vi "ControlRefnumStore__slk_refnum.vi"(6 "cmd (Get)":enum16{"Set", "Get"}(ring)=enum."Get", 8 "error in (no error)":errorcluster, 11 "vi refnum in (use current vi if non-wired)":refnum<vi>) -> (0 "error out":errorcluster, 3 "control refnum array out":refnum<vi>[](array[refnum]))   [LabVIEW 2020, in "REFNUM.lvlib"]
doc: "<b>Refnum Functions:</b>\nReset - Initializes all controls' refnum from current VI to GL.\nGet - Gets all controls's refnum from GL."
uses:
  Library/Refnum.lvlib
panel:
  # "ControlRefnumStore__slk_refnum.vi\n\nNOTICE -- YOU MUST LEAVE THIS NOTICE IN PLACE.\n\nCopyright (c) 2008 Shawn Liu <shawn.liu.cn@gmail.com>\n\nAll rights reserved."
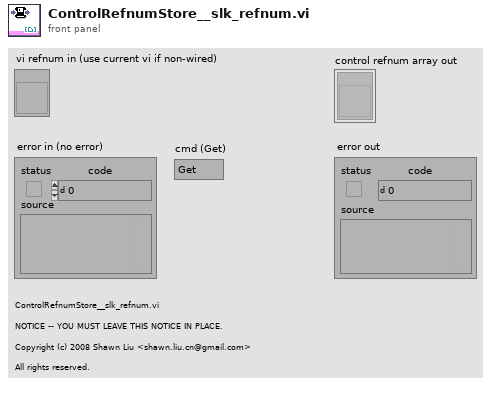
[diagram p1: front panel]
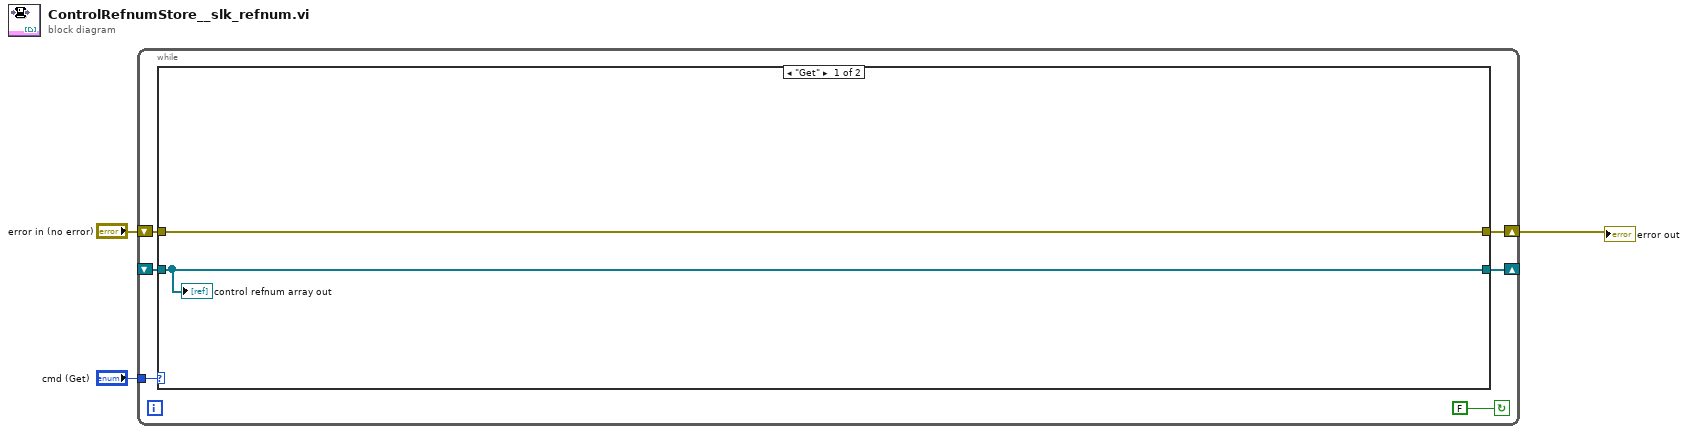
[diagram p0: block diagram]
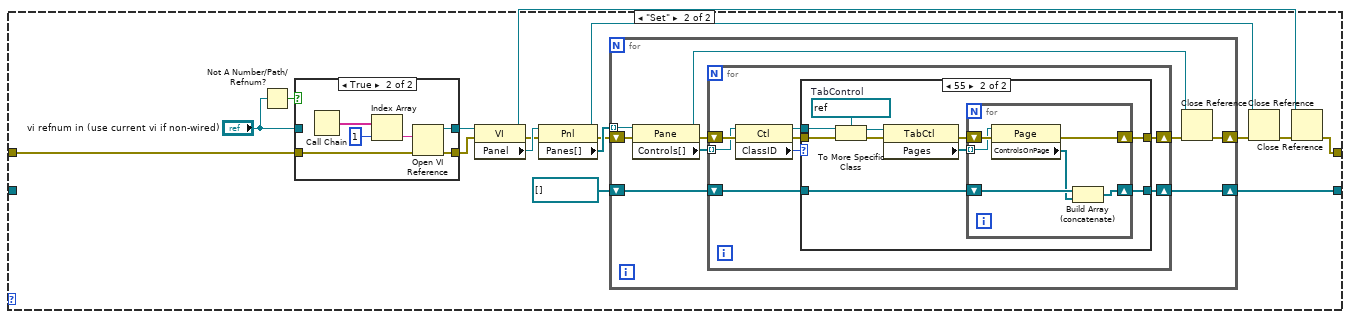
[diagram p2: hidden frame]
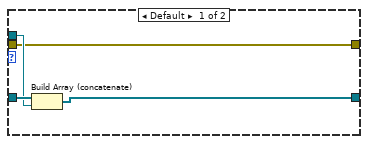
[diagram p4: hidden frame]
diagram:
  n1 = while {
    tunnel: "cmd (Get)" -> [w9]
    shift-right: [w8] -> _
    shift-left: _ -> [w7]
    shift-right: [w5] -> w1
    shift-left: "error in (no error)" -> [w6]
    stop <- FALSE continue-if-true
    n2 = case shown="\"Get\"" w9 {
      tunnel: [w11 w25] -> w8
      tunnel: w7 -> [w11 _]
      tunnel: w6 -> [w10 w21]
      tunnel: [w10 w24] -> w5
      frame "Get" {
        "control refnum array out" <- w11
      }
      frame "Set" {
        n3 = Not A Number/Path/Refnum?(number/path/refnum="vi refnum in (use current vi if non-wired)") -> (NaN/Path/Refnum?=w23:bool)
        n4 = case shown="True" w23 {
          tunnel: [w29 w32] -> w19
          tunnel: [w28 w31] -> w20
          tunnel: w21 -> [w28 w30]
          tunnel: "vi refnum in (use current vi if non-wired)" -> [w29 _]
          frame False {
          }
          frame True {
            n5 = Call Chain() -> (call chain=w35:string[])
            n6 = Index Array(array=w35, index=1) -> (element=w33:string)
            n7 = Open VI Reference(vi path=w33, error in (no error)=w30) -> (vi reference=w32:refnum<vi>, error out=w31:errorcluster)  [unwired: 4 out]
          }
        }
        n8 = property class="VI"(reference=w19, error in=w20) -> (reference out=w12:refnum<vi>, error out=w17:errorcluster, "Panel"=w18:refnum<vi>)
        n9 = property class="Pnl"(reference=w18, error in=w17) -> (reference out=w13:refnum<vi>, error out=w15:errorcluster, "Panes[]"=w16:refnum<vi>[])
        n10 = for {
          tunnel: w16 -> [w44] mode=indexing
          shift-right: [w37] -> w14
          shift-left: w15 -> [w43]
          shift-right: [w41] -> w25
          shift-left: refnum<vi>[] [] -> [w42]
          n11 = property class="Pane"(reference=w44, error in=w43) -> (reference out=w36:refnum<vi>, error out=w39:errorcluster, "Controls[]"=w40:refnum<vi>[])
          n12 = for {
            shift-right: [w45] -> w41
            shift-left: w42 -> [w47]
            tunnel: w40 -> [w51] mode=indexing
            shift-right: [w46] -> w38
            shift-left: w39 -> [w52]
            n13 = property class="Ctl"(reference=w51, error in=w52) -> (reference out=w49:refnum<vi>, error out=w48:errorcluster, "ClassID"=w50:u32)
            n14 = case shown="55" w50 {
              tunnel: w49 -> [w54 w64]
              tunnel: w48 -> [w53 w66]
              tunnel: w47 -> [w56 w59]
              tunnel: [w53 w58] -> w46
              tunnel: [w55 w57] -> w45
              frame Default {
                n15 = Build Array (concatenate)(w56, w54) -> (w55:refnum<vi>[])
              }
              frame 55 {
                w62 = refnum<vi> refnum  # TabControl
                n16 = To More Specific Class(target class=w62, reference=w64, error in=w66) -> (specific class reference=w63:refnum<vi>, error out=w65:errorcluster)
                n17 = property class="TabCtl"(reference=w63, error in=w65) -> (error out=w60:errorcluster, "Pages"=w61:refnum<vi>[])  [unwired: 1 out]
                n18 = for {
                  tunnel: w61 -> [w71] mode=indexing
                  shift-right: [w68] -> w57
                  shift-left: w59 -> [w70]
                  shift-right: [w67] -> w58
                  shift-left: w60 -> [w72]
                  n19 = property class="Page"(reference=w71, error in=w72) -> (error out=w67:errorcluster, "ControlsOnPage"=w69:refnum<vi>[])  [unwired: 1 out]
                  n20 = Build Array (concatenate)(w70, w69) -> (w68:refnum<vi>[])
                }
              }
            }
          }
          n21 = Close Reference(reference=w36, error in (no error)=w38) -> (error out=w37:errorcluster)
        }
        n22 = Close Reference(reference=w13, error in (no error)=w14) -> (error out=w26:errorcluster)
        n23 = Close Reference(reference=w12, error in (no error)=w26) -> (error out=w24:errorcluster)
      }
    }
  }
  "error out" <- w1
